vi "Launch Shutdown Optimization.vi"(8 "error in":errorcluster, 11 "SCADA in":refnum<class "EMS.lvclass">) -> (0 "error out":errorcluster, 3 "SCADA out":refnum<class "EMS.lvclass">)   [LabVIEW 2018, in "EMS Core.lvlib" / "EMS.lvclass"]
uses:
  EMS.lvclass
  C:/Users/Administrator/Desktop/LabVIEW EMS/EMS Generic Actor/EMS Generic/EMS Generic.lvclass
  C:/Program Files (x86)/National Instruments/LabVIEW 2018/vi.lib/ActorFramework/Actor/Actor.lvclass
  Optimization/Shutdown Actor/Shutdown/Shutdown.lvclass
  C:/Users/Administrator/Desktop/LabVIEW EMS/Device Communication and Control Abstract Actor/Device Communication and Control Abstract/Device Communication and Control Abstract.lvclass
  C:/Users/Administrator/Desktop/LabVIEW EMS/Optimization/Generic Optimization Actor/Generic Optimization/Generic Optimization.lvclass
  EMS Messages/Shutdown Complete Msg/Shutdown Complete Msg.lvclass
  C:/Users/Administrator/Desktop/LabVIEW EMS/Optimization/Generic Optimization Actor/Generic Optimization Messages/Operation Complete Msg/Operation Complete Msg.lvclass
  Optimization/Generic Optimization Actor/Generic Optimization/Generic Optimization.lvclass/Generic Optimization.ctl
  EMS.lvclass/EMS.ctl
  <vilib>/ActorFramework/Actor/Actor.lvclass
  Optimization/Generic Optimization Actor/Generic Optimization/Generic Optimization.lvclass
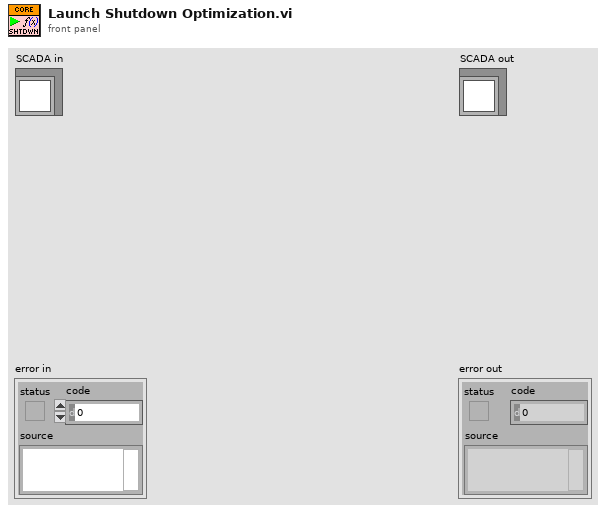
[diagram p1: front panel]
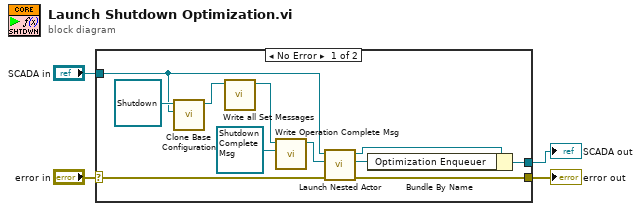
[diagram p0: block diagram]
diagram:
  n1 = case shown="No Error" "error in" {
    selector: "error in" -> [w8 w17]
    tunnel: [w14 w17] -> w3
    tunnel: [w13 w16] -> w1
    tunnel: "SCADA in" -> [w5 w16]
    frame No Error {
      n2 = call-dynamic "Clone Base Configuration.vi"("Source Object"=w5, "Target Object in"=refnum<class "Shutdown.lvclass"> refnum ("Shutdown Actor.lvlib:Shutdown.lvclass")) -> ("Target Object out"=w6:refnum<class "Shutdown.lvclass">)  [unwired: 9 in]
      n3 = call "Write all Set Messages.vi"("Device Communication and Control Abstract In"=w6) -> ("Device Communication and Control Abstract Out"=w11:refnum<class "Shutdown.lvclass">)  [unwired: 10 in]
      n4 = call "Write Operation Complete Msg.vi"("Operation Complete Msg"=refnum<class "Shutdown Complete Msg.lvclass"> refnum ("SCADA Core.lvlib:Shutdown Complete Msg.lvclass"), "Generic Optimization in"=w11) -> ("Generic Optimization out"=w10:refnum<class "Shutdown.lvclass">)  [unwired: 9 in]
      n5 = call <vilib>:"Launch Nested Actor.vi"("error in (no error)"=w8, "Nested Actor"=w10, "Caller Actor in"=w5) -> ("error out"=w14:errorcluster, "Nested Actor's Enqueuer"=w12:refnum<class "Message Enqueuer.lvclass">, "Caller Actor out"=w15:refnum<class "EMS.lvclass">)  [unwired: 6 in]
      n6 = Bundle By Name(cluster=w15, "Optimization Enqueuer"=w12) -> (w13:refnum<class "EMS.lvclass">)
    }
    frame Error {
    }
  }
  "error out" <- w3
  "SCADA out" <- w1
